vi "Send Emergency Stop.vi"(8 "error in (no error)":errorcluster, 11 "Message Enqueuer":refnum<class "Message Enqueuer.lvclass">) -> (0 "error out":errorcluster)   [LabVIEW 2017, in "Actor Framework.lvlib" / "Stop Msg.lvclass"]
doc: "(<B>Filename</B>: Actor Framework.lvlib:Stop Msg.lvclass:Send Emergency Stop.vi)\n\nSends an Emergency Stop message to an actor, triggering the actor to shut down as quickly as possible. This message has critical priority, meaning it will be processed before all messages that are already in the queue."
uses:
  <vilib>/ActorFramework/Stop Msg/Stop Msg.lvclass
  <vilib>/ActorFramework/Message Enqueuer/Message Enqueuer.lvclass
  e:/builds/penguin/labview/branches/2017/dev/dist/vi.lib/ActorFramework/Message/Message.lvclass
  <vilib>/ActorFramework/Stop Msg/Stop Msg.lvclass/Stop Msg.ctl
  <vilib>/ActorFramework/Message Enqueuer/Message Enqueuer.lvclass/Message Enqueuer.ctl
  <vilib>/ActorFramework/Message Priority Queue/Priority Enqueue.vi
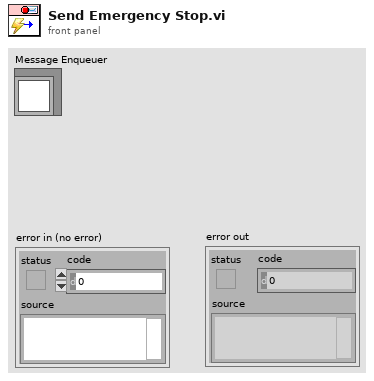
[diagram p1: front panel]
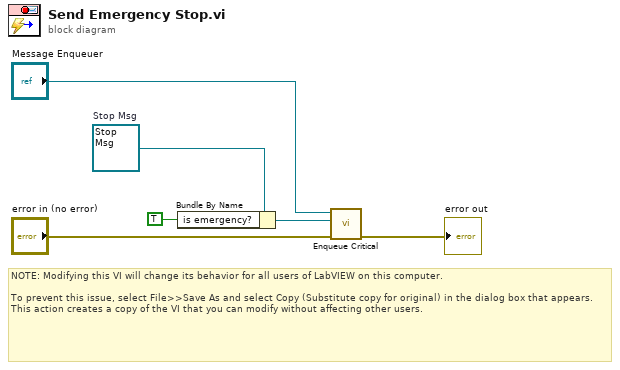
[diagram p0: block diagram]
diagram:
  w6 = refnum<class "Stop Msg.lvclass"> refnum  # Stop Msg
  # "NOTE: Modifying this VI will change its behavior for all users of LabVIEW on this computer.\n\nTo prevent this issue, select File>>Save As and select Copy (Substitute copy for original) in the dialog box that appears. This action creates a copy of the VI that you can modify without affecting other users."
  n1 = Bundle By Name(cluster=w6, "is emergency?"=TRUE) -> (w3:refnum<class "Stop Msg.lvclass">)
  n2 = call <vilib>:"Enqueue Critical.vi"("error in (no error)"="error in (no error)", "Message"=w3, "Message Enqueuer in"="Message Enqueuer") -> ("error out"=→"error out":errorcluster)  [unwired: 7 in, 1 out]
